vi "LorentzianWithFilter.vi"(3 "output control":T1, 4 "data":T2, 5 "X":dbl[](array[numeric]), 6 "a":dbl[](array[numeric])) -> (0 "error out":errorcluster, 1 "f'(X,a)":dbl[][](array[numeric]), 2 "f(X,a)":dbl[](array[numeric]))   [LabVIEW 2010]
doc: "This template is the starting point for creating a model function to be passed to the Nonlinear Curve Fit.vi."
uses:
  <vilib>/gmath/NumericalOptimization/objective function data.ctl
  <vilib>/gmath/NumericalOptimization/LM_output select.ctl
  <vilib>/gmath/NI_Gmath.lvlib
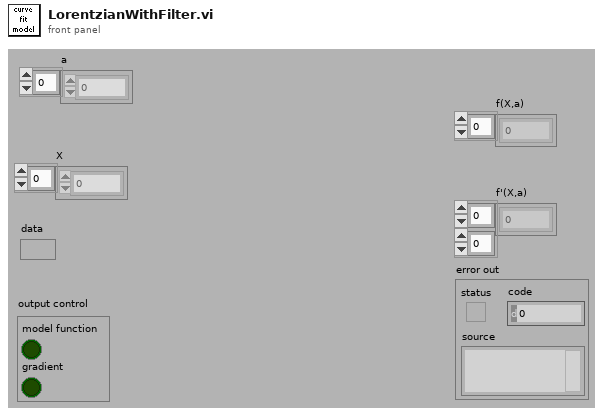
[diagram p1: front panel]
types:
  T1 = typedef "NI_Gmath.lvlib/LM_output select.ctl" = cluster{"model function":bool, "gradient":bool}
  T2 = typedef "NI_Gmath.lvlib/objective function data.ctl" = variant
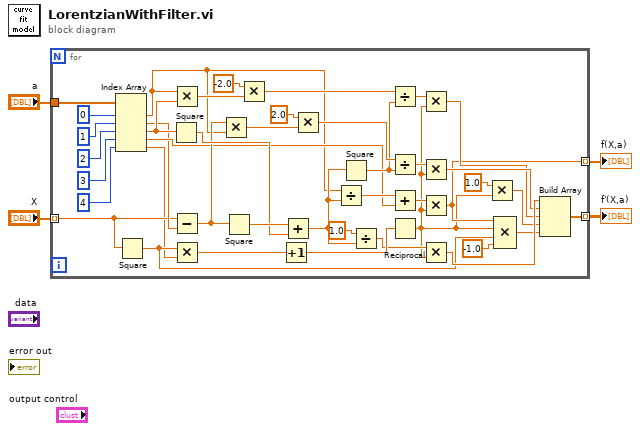
[diagram p0: block diagram]
diagram:
  n1 = for {
    tunnel: "a" -> [w46]
    tunnel: "X" -> [w23] mode=indexing
    tunnel: [w12] -> w2 mode=indexing
    tunnel: [w10] -> w1 mode=indexing
    n2 = Index Array(array=w46, index #1=0 ("index"), index #2=1 ("index"), index #3=2 ("index"), index #4=3 ("index"), index #5=4 ("index")) -> (element #1=w26:dbl, element #2=w25:dbl, element #3=w31:dbl, element #4=w32:dbl, element #5=w6:dbl)
    n3 = Square(x=w23) -> (x^2=w8:dbl)
    n4 = Square(x=w31) -> (x^2=w44:dbl)
    n5 = Multiply(x=w26, y=w31) -> (x*y=w35:dbl)
    n6 = Subtract(x=w23, y=w25) -> (x-y=w39:dbl)
    n7 = Multiply(x=w8, y=w6) -> (x*y=w22:dbl)
    n8 = Multiply(x=w39, y=w26) -> (x*y=w40:dbl)
    n9 = Square(x=w39) -> (x^2=w45:dbl)
    n10 = Multiply(x=-2.0, y=w35) -> (x*y=w34:dbl)
    n11 = Increment(x=w22) -> (x+1=w21:dbl)
    n12 = Add(x=w45, y=w44) -> (x+y=w37:dbl)
    n13 = Multiply(x=2.0, y=w40) -> (x*y=w38:dbl)
    n14 = Divide(x=w26, y=w37) -> (x/y=w43:dbl)
    n15 = Square(x=w37) -> (x^2=w33:dbl)
    n16 = Divide(x=1.0, y=w37) -> (x/y=w20:dbl)
    n17 = Divide(x=w34, y=w33) -> (x/y=w18:dbl)
    n18 = Divide(x=w38, y=w33) -> (x/y=w19:dbl)
    n19 = Add(x=w43, y=w32) -> (x+y=w11:dbl)
    n20 = Reciprocal(x=w21) -> (1/x=w9:dbl)
    n21 = Multiply(x=w18, y=w9) -> (x*y=w14:dbl)
    n22 = Multiply(x=w19, y=w9) -> (x*y=w15:dbl)
    n23 = Multiply(x=w11, y=w9) -> (x*y=w10:dbl)
    n24 = Multiply(x=w20, y=w9) -> (x*y=w16:dbl)
    n25 = Multiply(x=1.0, y=w9) -> (x*y=w13:dbl)
    n26 = Compound Arithmetic op=MULTIPLY(w10, w9, w8, -1.0 ("value")) -> (w7:dbl)
    n27 = Build Array(w16, w15, w14, w13, w7) -> (w12:dbl[])
  }
  "f(X,a)" <- w1
  "f'(X,a)" <- w2
